vi "InitImageDisplay.vi"(8 "error in (no error)":errorcluster) -> (0 "error out":errorcluster)   [LabVIEW 2017]
doc: "SciScan 1.2 160622"
uses:
  GFG/GFGImageRefsGet.vi
  GFG/GFGDisplayRefsGet.vi
  GFG/GFG library.lvlib
panel:
  out "Numeric Control":i32
  in  "?":u32(colorbox)=3618615
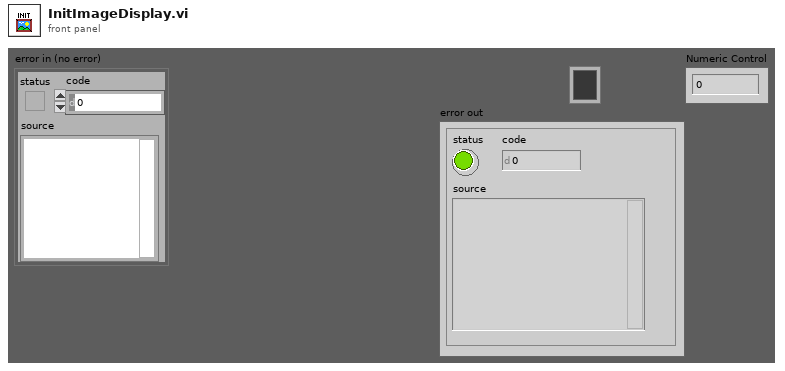
[diagram p1: front panel]
types:
  T1 = cluster{"Global Rectangle":i32[], "Contours":cluster{"Contour Type":u32, "ROI Type":u32, "Points":i32[]}[]}
  T2 = typedef "IMAQ Image.ctl" = refnum<image>
  T3 = cluster{"Channel 1 small":T2, "Channel 2 small":T2, "Channel 3 small":T2, "Channel 4 small":T2, "Channel 1 large":T2, "Channel 2 large":T2, "Channel 3 large":T2, "Channel 4 large":T2, "RGB overlay":T2, "ROI Image display":T2, "arb line scan display":T2, "Channel 5 large":T2}
  T4 = cluster{"Channel 1 small":refnum<vi>, "Channel 2 small":refnum<vi>, "Channel 3 small":refnum<vi>, "Channel 4 small":refnum<vi>, "Channel 1 large":refnum<vi>, "Channel 2 large":refnum<vi>, "Channel 3 large":refnum<vi>, "Channel 4 large":refnum<vi>, "RGB overlay":refnum<vi>, "ROI Image display":refnum<vi>, "arb line scan display":refnum<vi>, "Channel 5 large":refnum<vi>}
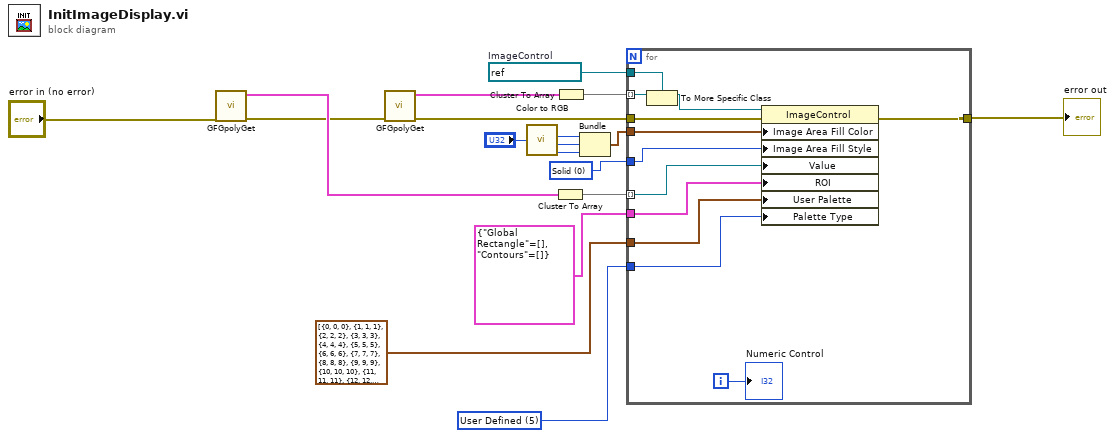
[diagram p0: block diagram]
diagram:
  w1 = u32 5 items=["Grayscale", "Binary", "Gradient", "Rainbow", "Temperature", "User Defined"] ("Palette:Palette Type")
  w9 = refnum<vi> refnum  # ImageControl
  w12 = u32 0 items=["Default"=3, "Solid"=0, "Hatch"=2] ("Image Area:Background:Fill Style")
  n1 = call-poly "GFGpolyGet.vi"("error in (no error)"="error in (no error)") -> ("error out"=w5:errorcluster, "Image Refs Out"=w8:T3)  [unwired: 9 in]
  n2 = call-poly "GFGpolyGet.vi"("error in (no error)"=w5) -> ("error out"=w4:errorcluster, "DisplayRefsOut(generic class)"=w7:T4)  [unwired: 9 in]
  n3 = call <vilib>:"Color to RGB.vi"("Color"="?") -> ("R"=w18:u8, "G"=w17:u8, "B"=w16:u8)  [unwired: 1 out]
  n4 = Cluster To Array(cluster=w8) -> (array=w11:T2[])
  n5 = Cluster To Array(cluster=w7) -> (array=w14:refnum<vi>[])
  n6 = Bundle("R"=w18, "G"=w17, "B"=w16) -> (w13:cluster{"R":u8, "G":u8, "B":u8})  [unwired: 1 in]
  n7 = for {
    tunnel: w14 -> [w25] mode=indexing
    tunnel: w13 -> [w30]
    tunnel: w12 -> [w29]
    tunnel: w11 -> [w28] mode=indexing
    tunnel: w4 -> [w27]
    tunnel: [w26] -> w10
    tunnel: w9 -> [w23]
    tunnel: T1 {"Global Rectangle"=[], "Contours"=[]} ("ROI") -> [w22]
    tunnel: cluster{"Red":u8, "Green":u8, "Blue":u8}[] [{"Red"=0, "Green"=0, "Blue"=0}, {"Red"=1, "Green"=1, "Blue"=1}, {"Red"=2, "Green"=2, "Blue"=2}, {"Red"=3, "Green"=3, "Blue"=3}, {"Red"=4, "Green"=4, "Blue"=4}, {"Red"=5, "Green"=5, "Blue"=5}, {"Red"=6, "Green"=6, "Blue"=6}, {"Red"=7, "Green"=7, "Blue"=7}, {"Red"=8, "Green"=8, "Blue"=8}, {"Red"=9, "Green"=9, "Blue"=9}, {"Red"=10, "Green"=10, "Blue"=10}, {"Red"=11, "Green"=11, "Blue"=11}, {"Red"=12, "Green"=12, "Blue"=12}, {"Red"=13, "Green"=13, "Blue"=13}, {"Red"=14, "Green"=14, "Blue"=14}, {"Red"=15, "Green"=15, "Blue"=15}, {"Red"=16, "Green"=16, "Blue"=16}, {"Red"=17, "Green"=17, "Blue"=17}, {"Red"=18, "Green"=18, "Blue"=18}, {"Red"=19, "Green"=19, "Blue"=19}, {"Red"=20, "Green"=20, "Blue"=20}, {"Red"=21, "Green"=21, "Blue"=21}, {"Red"=22, "Green"=22, "Blue"=22}, {"Red"=23, "Green"=23, "Blue"=23}, {"Red"=24, "Green"=24, "Blue"=24}, {"Red"=25, "Green"=25, "Blue"=25}, {"Red"=26, "Green"=26, "Blue"=26}, {"Red"=27, "Green"=27, "Blue"=27}, {"Red"=28, "Green"=28, "Blue"=28}, {"Red"=29, "Green"=29, "Blue"=29}, {"Red"=30, "Green"=30, "Blue"=30}, {"Red"=31, "Green"=31, "Blue"=31}, {"Red"=32, "Green"=32, "Blue"=32}, {"Red"=33, "Green"=33, "Blue"=33}, {"Red"=34, "Green"=34, "Blue"=34}, {"Red"=35, "Green"=35, "Blue"=35}, {"Red"=36, "Green"=36, "Blue"=36}, {"Red"=37, "Green"=37, "Blue"=37}, {"Red"=38, "Green"=38, "Blue"=38}, {"Red"=39, "Green"=39, "Blue"=39}, {"Red"=40, "Green"=40, "Blue"=40}, {"Red"=41, "Green"=41, "Blue"=41}, {"Red"=42, "Green"=42, "Blue"=42}, {"Red"=43, "Green"=43, "Blue"=43}, {"Red"=44, "Green"=44, "Blue"=44}, {"Red"=45, "Green"=45, "Blue"=45}, {"Red"=46, "Green"=46, "Blue"=46}, {"Red"=47, "Green"=47, "Blue"=47}, {"Red"=48, "Green"=48, "Blue"=48}, {"Red"=49, "Green"=49, "Blue"=49}, {"Red"=50, "Green"=50, "Blue"=50}, {"Red"=51, "Green"=51, "Blue"=51}, {"Red"=52, "Green"=52, "Blue"=52}, {"Red"=53, "Green"=53, "Blue"=53}, {"Red"=54, "Green"=54, "Blue"=54}, {"Red"=55, "Green"=55, "Blue"=55}, {"Red"=56, "Green"=56, "Blue"=56}, {"Red"=57, "Green"=57, "Blue"=57}, {"Red"=58, "Green"=58, "Blue"=58}, {"Red"=59, "Green"=59, "Blue"=59}, {"Red"=60, "Green"=60, "Blue"=60}, {"Red"=61, "Green"=61, "Blue"=61}, {"Red"=62, "Green"=62, "Blue"=62}, {"Red"=63, "Green"=63, "Blue"=63}, {"Red"=64, "Green"=64, "Blue"=64}, {"Red"=65, "Green"=65, "Blue"=65}, {"Red"=66, "Green"=66, "Blue"=66}, {"Red"=67, "Green"=67, "Blue"=67}, {"Red"=68, "Green"=68, "Blue"=68}, {"Red"=69, "Green"=69, "Blue"=69}, {"Red"=70, "Green"=70, "Blue"=70}, {"Red"=71, "Green"=71, "Blue"=71}, {"Red"=72, "Green"=72, "Blue"=72}, {"Red"=73, "Green"=73, "Blue"=73}, {"Red"=74, "Green"=74, "Blue"=74}, {"Red"=75, "Green"=75, "Blue"=75}, {"Red"=76, "Green"=76, "Blue"=76}, {"Red"=77, "Green"=77, "Blue"=77}, {"Red"=78, "Green"=78, "Blue"=78}, {"Red"=79, "Green"=79, "Blue"=79}, {"Red"=80, "Green"=80, "Blue"=80}, {"Red"=81, "Green"=81, "Blue"=81}, {"Red"=82, "Green"=82, "Blue"=82}, {"Red"=83, "Green"=83, "Blue"=83}, {"Red"=84, "Green"=84, "Blue"=84}, {"Red"=85, "Green"=85, "Blue"=85}, {"Red"=86, "Green"=86, "Blue"=86}, {"Red"=87, "Green"=87, "Blue"=87}, {"Red"=88, "Green"=88, "Blue"=88}, {"Red"=89, "Green"=89, "Blue"=89}, {"Red"=90, "Green"=90, "Blue"=90}, {"Red"=91, "Green"=91, "Blue"=91}, {"Red"=92, "Green"=92, "Blue"=92}, {"Red"=93, "Green"=93, "Blue"=93}, {"Red"=94, "Green"=94, "Blue"=94}, {"Red"=95, "Green"=95, "Blue"=95}, {"Red"=96, "Green"=96, "Blue"=96}, {"Red"=97, "Green"=97, "Blue"=97}, {"Red"=98, "Green"=98, "Blue"=98}, {"Red"=99, "Green"=99, "Blue"=99}, {"Red"=100, "Green"=100, "Blue"=100}, {"Red"=101, "Green"=101, "Blue"=101}, {"Red"=102, "Green"=102, "Blue"=102}, {"Red"=103, "Green"=103, "Blue"=103}, {"Red"=104, "Green"=104, "Blue"=104}, {"Red"=105, "Green"=105, "Blue"=105}, {"Red"=106, "Green"=106, "Blue"=106}, {"Red"=107, "Green"=107, "Blue"=107}, {"Red"=108, "Green"=108, "Blue"=108}, {"Red"=109, "Green"=109, "Blue"=109}, {"Red"=110, "Green"=110, "Blue"=110}, {"Red"=111, "Green"=111, "Blue"=111}, {"Red"=112, "Green"=112, "Blue"=112}, {"Red"=113, "Green"=113, "Blue"=113}, {"Red"=114, "Green"=114, "Blue"=114}, {"Red"=115, "Green"=115, "Blue"=115}, {"Red"=116, "Green"=116, "Blue"=116}, {"Red"=117, "Green"=117, "Blue"=117}, {"Red"=118, "Green"=118, "Blue"=118}, {"Red"=119, "Green"=119, "Blue"=119}, {"Red"=120, "Green"=120, "Blue"=120}, {"Red"=121, "Green"=121, "Blue"=121}, {"Red"=122, "Green"=122, "Blue"=122}, {"Red"=123, "Green"=123, "Blue"=123}, {"Red"=124, "Green"=124, "Blue"=124}, {"Red"=125, "Green"=125, "Blue"=125}, {"Red"=126, "Green"=126, "Blue"=126}, {"Red"=127, "Green"=127, "Blue"=127}, {"Red"=128, "Green"=128, "Blue"=128}, {"Red"=129, "Green"=129, "Blue"=129}, {"Red"=130, "Green"=130, "Blue"=130}, {"Red"=131, "Green"=131, "Blue"=131}, {"Red"=132, "Green"=132, "Blue"=132}, {"Red"=133, "Green"=133, "Blue"=133}, {"Red"=134, "Green"=134, "Blue"=134}, {"Red"=135, "Green"=135, "Blue"=135}, {"Red"=136, "Green"=136, "Blue"=136}, {"Red"=137, "Green"=137, "Blue"=137}, {"Red"=138, "Green"=138, "Blue"=138}, {"Red"=139, "Green"=139, "Blue"=139}, {"Red"=140, "Green"=140, "Blue"=140}, {"Red"=141, "Green"=141, "Blue"=141}, {"Red"=142, "Green"=142, "Blue"=142}, {"Red"=143, "Green"=143, "Blue"=143}, {"Red"=144, "Green"=144, "Blue"=144}, {"Red"=145, "Green"=145, "Blue"=145}, {"Red"=146, "Green"=146, "Blue"=146}, {"Red"=147, "Green"=147, "Blue"=147}, {"Red"=148, "Green"=148, "Blue"=148}, {"Red"=149, "Green"=149, "Blue"=149}, {"Red"=150, "Green"=150, "Blue"=150}, {"Red"=151, "Green"=151, "Blue"=151}, {"Red"=152, "Green"=152, "Blue"=152}, {"Red"=153, "Green"=153, "Blue"=153}, {"Red"=154, "Green"=154, "Blue"=154}, {"Red"=155, "Green"=155, "Blue"=155}, {"Red"=156, "Green"=156, "Blue"=156}, {"Red"=157, "Green"=157, "Blue"=157}, {"Red"=158, "Green"=158, "Blue"=158}, {"Red"=159, "Green"=159, "Blue"=159}, {"Red"=160, "Green"=160, "Blue"=160}, {"Red"=161, "Green"=161, "Blue"=161}, {"Red"=162, "Green"=162, "Blue"=162}, {"Red"=163, "Green"=163, "Blue"=163}, {"Red"=164, "Green"=164, "Blue"=164}, {"Red"=165, "Green"=165, "Blue"=165}, {"Red"=166, "Green"=166, "Blue"=166}, {"Red"=167, "Green"=167, "Blue"=167}, {"Red"=168, "Green"=168, "Blue"=168}, {"Red"=169, "Green"=169, "Blue"=169}, {"Red"=170, "Green"=170, "Blue"=170}, {"Red"=171, "Green"=171, "Blue"=171}, {"Red"=172, "Green"=172, "Blue"=172}, {"Red"=173, "Green"=173, "Blue"=173}, {"Red"=174, "Green"=174, "Blue"=174}, {"Red"=175, "Green"=175, "Blue"=175}, {"Red"=176, "Green"=176, "Blue"=176}, {"Red"=177, "Green"=177, "Blue"=177}, {"Red"=178, "Green"=178, "Blue"=178}, {"Red"=179, "Green"=179, "Blue"=179}, {"Red"=180, "Green"=180, "Blue"=180}, {"Red"=181, "Green"=181, "Blue"=181}, {"Red"=182, "Green"=182, "Blue"=182}, {"Red"=183, "Green"=183, "Blue"=183}, {"Red"=184, "Green"=184, "Blue"=184}, {"Red"=185, "Green"=185, "Blue"=185}, {"Red"=186, "Green"=186, "Blue"=186}, {"Red"=187, "Green"=187, "Blue"=187}, {"Red"=188, "Green"=188, "Blue"=188}, {"Red"=189, "Green"=189, "Blue"=189}, {"Red"=190, "Green"=190, "Blue"=190}, {"Red"=191, "Green"=191, "Blue"=191}, {"Red"=192, "Green"=192, "Blue"=192}, {"Red"=193, "Green"=193, "Blue"=193}, {"Red"=194, "Green"=194, "Blue"=194}, {"Red"=195, "Green"=195, "Blue"=195}, {"Red"=196, "Green"=196, "Blue"=196}, {"Red"=197, "Green"=197, "Blue"=197}, {"Red"=198, "Green"=198, "Blue"=198}, {"Red"=199, "Green"=199, "Blue"=199}, {"Red"=200, "Green"=200, "Blue"=200}, {"Red"=201, "Green"=201, "Blue"=201}, {"Red"=202, "Green"=202, "Blue"=202}, {"Red"=203, "Green"=203, "Blue"=203}, {"Red"=204, "Green"=204, "Blue"=204}, {"Red"=205, "Green"=205, "Blue"=205}, {"Red"=206, "Green"=206, "Blue"=206}, {"Red"=207, "Green"=207, "Blue"=207}, {"Red"=208, "Green"=208, "Blue"=208}, {"Red"=209, "Green"=209, "Blue"=209}, {"Red"=210, "Green"=210, "Blue"=210}, {"Red"=211, "Green"=211, "Blue"=211}, {"Red"=212, "Green"=212, "Blue"=212}, {"Red"=213, "Green"=213, "Blue"=213}, {"Red"=214, "Green"=214, "Blue"=214}, {"Red"=215, "Green"=215, "Blue"=215}, {"Red"=216, "Green"=216, "Blue"=216}, {"Red"=217, "Green"=217, "Blue"=217}, {"Red"=218, "Green"=218, "Blue"=218}, {"Red"=219, "Green"=219, "Blue"=219}, {"Red"=220, "Green"=220, "Blue"=220}, {"Red"=221, "Green"=221, "Blue"=221}, {"Red"=222, "Green"=222, "Blue"=222}, {"Red"=223, "Green"=223, "Blue"=223}, {"Red"=224, "Green"=224, "Blue"=224}, {"Red"=225, "Green"=225, "Blue"=225}, {"Red"=226, "Green"=226, "Blue"=226}, {"Red"=227, "Green"=227, "Blue"=227}, {"Red"=228, "Green"=228, "Blue"=228}, {"Red"=229, "Green"=229, "Blue"=229}, {"Red"=230, "Green"=230, "Blue"=230}, {"Red"=231, "Green"=231, "Blue"=231}, {"Red"=232, "Green"=232, "Blue"=232}, {"Red"=233, "Green"=233, "Blue"=233}, {"Red"=234, "Green"=234, "Blue"=234}, {"Red"=235, "Green"=235, "Blue"=235}, {"Red"=236, "Green"=236, "Blue"=236}, {"Red"=237, "Green"=237, "Blue"=237}, {"Red"=238, "Green"=238, "Blue"=238}, {"Red"=239, "Green"=239, "Blue"=239}, {"Red"=240, "Green"=240, "Blue"=240}, {"Red"=241, "Green"=241, "Blue"=241}, {"Red"=242, "Green"=242, "Blue"=242}, {"Red"=243, "Green"=243, "Blue"=243}, {"Red"=244, "Green"=244, "Blue"=244}, {"Red"=245, "Green"=245, "Blue"=245}, {"Red"=246, "Green"=246, "Blue"=246}, {"Red"=247, "Green"=247, "Blue"=247}, {"Red"=248, "Green"=248, "Blue"=248}, {"Red"=249, "Green"=249, "Blue"=249}, {"Red"=250, "Green"=250, "Blue"=250}, {"Red"=251, "Green"=251, "Blue"=251}, {"Red"=252, "Green"=252, "Blue"=252}, {"Red"=253, "Green"=253, "Blue"=253}, {"Red"=254, "Green"=254, "Blue"=254}, {"Red"=255, "Green"=255, "Blue"=255}] ("Color Palette") -> [w21]
    tunnel: w1 -> [w20]
    i -> [w19]
    n8 = To More Specific Class(target class=w23, reference=w25) -> (specific class reference=w24:refnum<vi>)  [unwired: 1 in, 1 out]
    n9 = property class="ImageControl"(reference=w24, error in=w27, "Image Area Fill Color"=w30, "Image Area Fill Style"=w29, "Value"=w28, "ROI"=w22, "User Palette"=w21, "Palette Type"=w20) -> (error out=w26:errorcluster)  [unwired: 1 out]
    "Numeric Control" <- w19
  }
  "error out" <- w10
